vi "User_Table_Update.vi"(7 "Last_User_Name":string, 8 "error in (no error)":errorcluster caption="错误输入（无错误）", 9 "Password":string, 10 "User_Right":u16(ring) caption="权    限" items=["操作员"=2], 11 "Name":string) -> (0 "error out":errorcluster caption="错误输出")   [LabVIEW 2020]
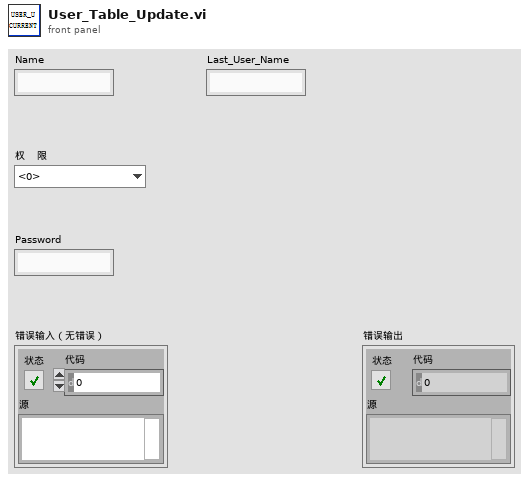
[diagram p1: front panel]
types:
  T1 = cluster{"Name":string, "User_Right":u16, "Password":string}
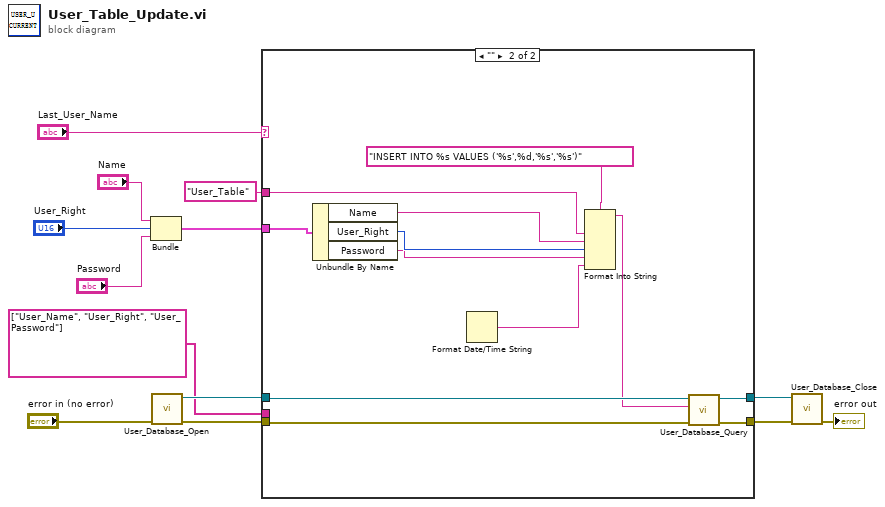
[diagram p0: block diagram]
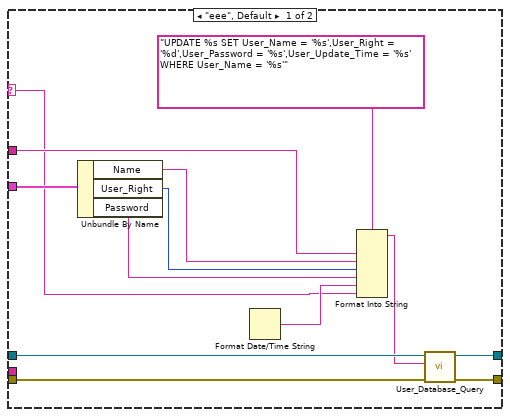
[diagram p2: hidden frame]
diagram:
  n1 = Bundle("Name"="Name", "User_Right"="User_Right", "Password"="Password") -> (w5:T1)  [unwired: 1 in]
  n2 = call "User_Database_Open.vi"("error in (no error)"="error in (no error)") -> ("error out"=w8:errorcluster, "SQLite Connection"=w9:refnum<class "Connection.lvclass">)  [unwired: 9 in]
  n3 = case shown="\"\"" "Last_User_Name" {
    selector: "Last_User_Name" -> [w14 _]
    tunnel: w9 -> [w26 w35]
    tunnel: w8 -> [w25 w38]
    tunnel: [w24 w37] -> w7
    tunnel: [w23 w36] -> w6
    tunnel: w5 -> [w20 w32]
    tunnel: string[] ["User_Name", "User_Right", "User_Password"] -> [_ _]
    tunnel: "User_Table" ("table") -> [w21 w33]
    frame "eee", Default {
      n4 = Unbundle By Name(w20) -> ("Name"=w17:string, "User_Right"=w19:u16, "Password"=w16:string)
      n5 = Format Date/Time String() -> (date/time string=w15:string)  [unwired: 3 in]
      n6 = Format Into String(format string="UPDATE %s SET User_Name = '%s',User_Right = '%d',User_Password = '%s',User_Update_Time = '%s' WHERE User_Name = '%s'" ("condition"), w21, w17, w19, w16, w15, w14) -> (resulting string=w18:string)  [unwired: 2 in, 1 out]
      n7 = call "User_Database_Query.vi"("error in (no error)"=w25, "SQL query"=w18, "SQLite Connection in"=w26) -> ("error out"=w24:errorcluster, "SQLite Connection"=w23:refnum<class "Connection.lvclass">)  [unwired: 6 in, 1 out]
    }
    frame "" {
      n8 = Unbundle By Name(w32) -> ("Name"=w31:string, "User_Right"=w30:u16, "Password"=w29:string)
      n9 = Format Date/Time String() -> (date/time string=w28:string)  [unwired: 3 in]
      n10 = Format Into String(format string="INSERT INTO %s VALUES ('%s',%d,'%s','%s')" ("condition"), w33, w31, w30, w29, w28) -> (resulting string=w27:string)  [unwired: 2 in, 1 out]
      n11 = call "User_Database_Query.vi"("error in (no error)"=w38, "SQL query"=w27, "SQLite Connection in"=w35) -> ("error out"=w37:errorcluster, "SQLite Connection"=w36:refnum<class "Connection.lvclass">)  [unwired: 6 in, 1 out]
    }
  }
  n12 = call "User_Database_Close.vi"("error in (no error)"=w7, "SQLite Connection in"=w6) -> ("error out"=→"error out":errorcluster)  [unwired: 9 in]
